vi "Empty Cluster.vi"() -> (0 "Empty Cluster":variant)   [LabVIEW 2019, in "JKI JSON Serialization.lvlib"]
doc: "JKI JSON 1.1.10.37\nTomi Maila - JKI\nCopyright (c) 2017, JKI"
uses:
  JKI JSON Serialization.lvlib
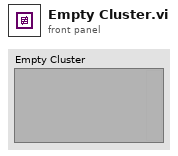
[diagram p1: front panel]
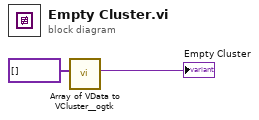
[diagram p0: block diagram]
diagram:
  n1 = call "Array of VData to VCluster__ogtk.vi"("Array"=variant[] []) -> ("VCluster"=→"Empty Cluster":variant)  [unwired: 9 in, 1 out]
